vi "update peak anott. colour.vi"(7 "Color":u32(colorbox), 8 "error in":errorcluster, 9 "Number of peak anott.":i32, 10 "starting index":i32, 11 "XY Graph":refnum<vi>) -> (0 "error out":errorcluster, 3 "XY Graph out":refnum<vi>)   [LabVIEW 2014]
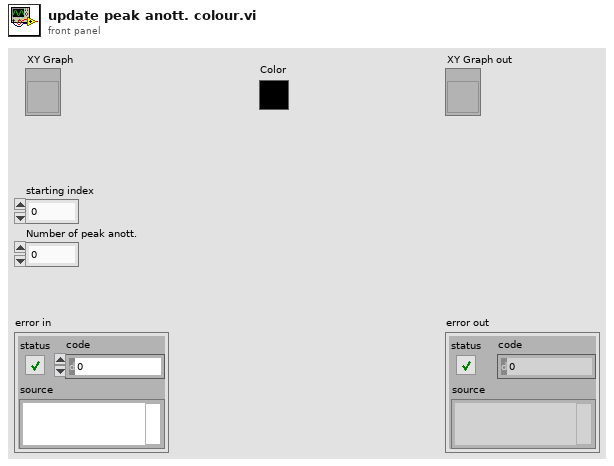
[diagram p1: front panel]
types:
  T1 = typedef "LVAnnotationListTypeDef.ctl" = cluster{"Name":string, "Color":u32, "Style":u8, "Point Style":u8, "Name Visible":bool, "Allow Drag":bool, "Annotation Mode":u32, "Plot":i32, "Index":i32, "Position":cluster{"X":dbl, "Y":dbl}, "X Scale":u32, "Y Scale":u32, "Show Arrow":bool, "Lock Name":bool, "Plot Area":i32, "Label Offset":cluster{"X":dbl, "Y":dbl}}[]
  T2 = cluster{"Name":string, "Color":u32, "Style":u8, "Point Style":u8, "Name Visible":bool, "Allow Drag":bool, "Annotation Mode":u32, "Plot":i32, "Index":i32, "Position":cluster{"X":dbl, "Y":dbl}, "X Scale":u32, "Y Scale":u32, "Show Arrow":bool, "Lock Name":bool, "Plot Area":i32, "Label Offset":cluster{"X":dbl, "Y":dbl}}
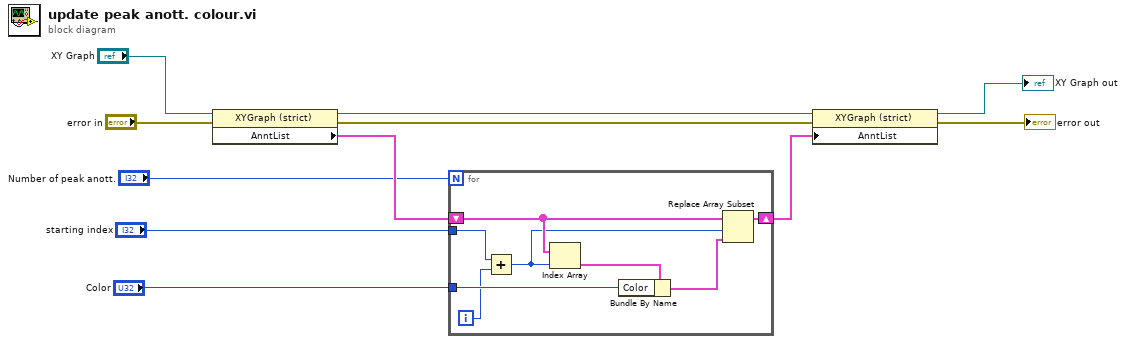
[diagram p0: block diagram]
diagram:
  n1 = property class="XYGraph (strict)"(reference="XY Graph", error in="error in") -> (reference out=w10:refnum<vi>, error out=w6:errorcluster, "AnntList"=w8:T1)
  n2 = for {
    N: "Number of peak anott." -> [_]
    tunnel: "Color" -> [w18]
    tunnel: "starting index" -> [w13]
    shift-right: [w15] -> w5
    shift-left: w8 -> [w17]
    i -> [w14]
    n3 = Add(x=w13, y=w14) -> (x+y=w12:i32)
    n4 = Index Array(array=w17, index=w12) -> (element=w19:T2)
    n5 = Bundle By Name(cluster=w19, "Color"=w18) -> (w16:T2)
    n6 = Replace Array Subset(array=w17, new element=w16, index=w12) -> (w15:T1)
  }
  n7 = property class="XYGraph (strict)"(reference=w10, error in=w6, "AnntList"=w5) -> (reference out=→"XY Graph out":refnum<vi>, error out=→"error out":errorcluster)
